vi "MainRT.vi"() -> ()   [LabVIEW 2018]
uses:
  Type Defs/The Motion Parameters.ctl
  Type Defs/G Code Command Cluster.ctl
  <vilib>/Motion/Express/_s/nimc.ex.clearFaults.clearFaults.axis.vi
  <vilib>/Motion/Express/_s/nimc.ex.power.power.axis.vi
  <vilib>/Motion/Express/_s/nimc.ex.read.readFaults.axis.vi
  <vilib>/Motion/BlockNode/FB.NIMotion.xnode
panel:
  in  "G Code File Path":path=path "c:/ni-rt/1cmQube.gcode"
  out "Ready":bool
  out "G Code Parser Progress":dbl(slide) scale=0.0..1.0
  out "Current Extruder Temp":dbl
  out "Current Bed Temp":dbl
  in  "Set Bed Temp":dbl
  in  "Monitor Stop":bool
  out "G Code Command Cluster":T1
  out "Faults":i32[][](array[numeric])
  in  "Motion Parameters":T2={"Timeout"=-1.0, "Blend Mode"=10551335, "Acceleration"=50.0, "Deceleration"=50.0, "Accel. Jerk"=500.0, "Decel. Jerk"=500.0, "Smoothing"=1000.0, "Last Blend"=TRUE, "Blend Delay"=0.0} {"Blend Delay" format="%#_13g"; "Smoothing" format="%#_13g"; "Decel. Jerk" format="%#_13g"; "Accel. Jerk" format="%#_13g"; "Deceleration" format="%#_13g"; "Acceleration" format="%#_13g"; "Blend Mode" items=["At Profile Complete"=10551335, "At Deceleration"=10551334, "After Delay"=10551336]}
  out "Error Out":errorcluster
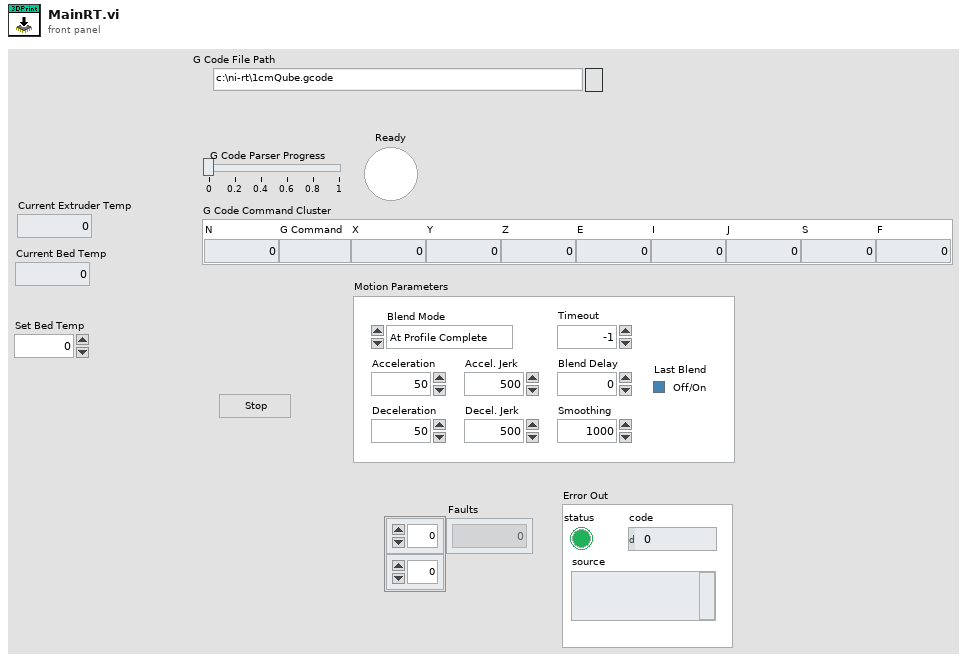
[diagram p1: front panel]
types:
  T1 = typedef "G Code Command Cluster.ctl" = cluster{"N":dbl, "G Command":string, "X":dbl, "Y":dbl, "Z":dbl, "E":dbl, "I":dbl, "J":dbl, "S":dbl, "F":dbl}
  T2 = typedef "The Motion Parameters.ctl" = cluster{"Timeout":dbl, "Blend Mode":i32, "Acceleration":dbl, "Deceleration":dbl, "Accel. Jerk":dbl, "Decel. Jerk":dbl, "Smoothing":dbl, "Last Blend":bool, "Blend Delay":dbl}
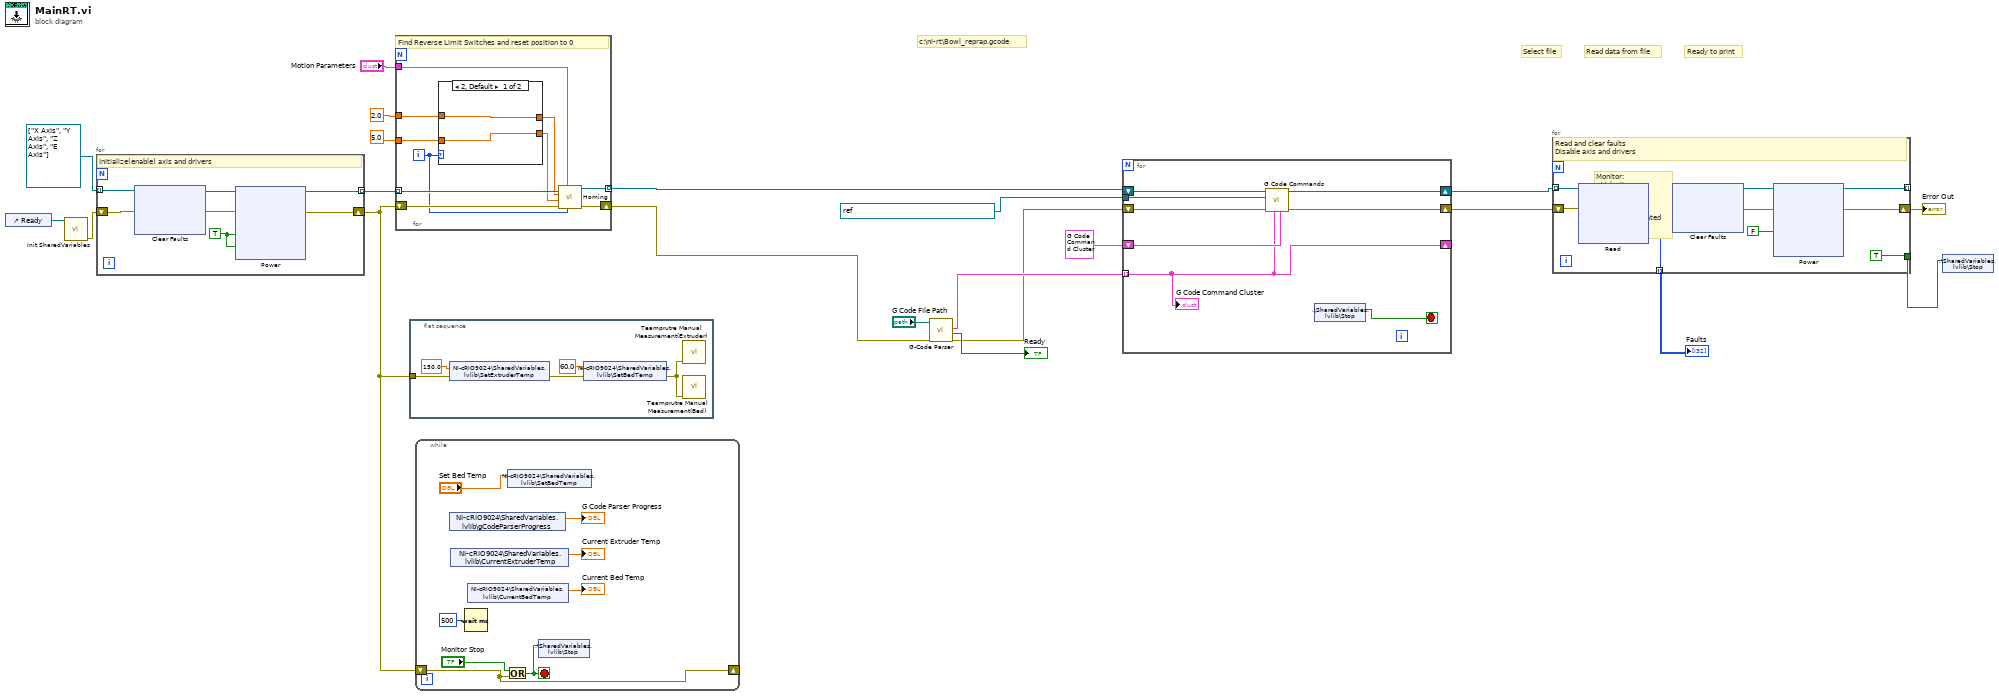
[diagram p0: block diagram]
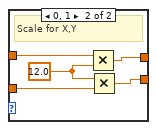
[diagram p2: hidden frame]
diagram:
  # "c:\\ni-rt\\Bowl_reprap.gcode"
  # "Ready to print"
  # "Select file"
  # "Monitor:\n- Velocity\n- Position\n- Faults\n- Temperature\n- Lines compleated"
  # "Execute G Code(for loop)"
  # "Read data from file"
  n1 = control-ref of="Ready"() -> (w1:refnum<vi>)
  n2 = call "Init SharedVariables.vi"("Boolean in"=w1) -> ("error out"=w4:errorcluster)  [unwired: 10 in]
  n3 = for {
    tunnel: refnum<k21>[] ["X Axis", "Y Axis", "Z Axis", "E Axis"] ("Axis Reference In") -> [w26] mode=indexing
    tunnel: [w25] -> w18 mode=indexing
    shift-right: [w23] -> w3
    shift-left: w4 -> [w22]
    w24 = TRUE ("enable axis")
    # "Initialize(enable) axis and drivers"
    n4 = xnode ("Clear Faults")("resource"=w26, "error in"=w22) -> ("resource out"=w28:refnum<k21>, "error out"=w27:errorcluster)
    n5 = xnode ("Power")("enable axis"=w24, "enable drive"=w24, "resource"=w28, "error in"=w27) -> ("resource out"=w25:refnum<k21>, "error out"=w23:errorcluster)
  }
  n6 = for {
    shift-right: [w49] -> w6
    shift-left: w3 -> [w50]
    tunnel: w18 -> [w48] mode=indexing
    tunnel: "Motion Parameters" -> [w44]
    tunnel: 5.0 ("Approach  Velocity") -> [w52]
    tunnel: 2.0 ("Search Velocity") -> [w51]
    tunnel: [w47] -> w5 mode=indexing
    i -> [w43]
    # "Find Reverse Limit Switches and reset position to 0"
    n7 = case shown="2, Default" w43 {
      tunnel: w52 -> [w54 w56]
      tunnel: [w54 w57] -> w46
      tunnel: w51 -> [w53 w58]
      tunnel: [w53 w59] -> w45
      frame 2, Default {
      }
      frame 0, 1 {
        w55 = 12.0 ("y")
        # "Scale for X,Y"
        n8 = Multiply(x=w58, y=w55) -> (x*y=w59:dbl)
        n9 = Multiply(x=w55, y=w56) -> (x*y=w57:dbl)
      }
    }
    n10 = call "Homing.vi"("Axis Index"=w43, "Motion Parameters"=w44, "Error In"=w50, "Approach  Velocity"=w46, "Search Velocity"=w45, "Axis Reference In"=w48) -> ("Error Out"=w49:errorcluster, "Axis Reference Out"=w47:refnum<k21>)  [unwired: 4 in]
  }
  n11 = flat-sequence {
    tunnel: w3 -> [w64]
    frame #0 {
      n12 = shared-variable "NI-cRIO9024\\SharedVariables.lvlib\\SetExtruderTemp"(150.0 ("Set Extruder Temp"), error in=w64) -> (error out=w63:errorcluster)
      n13 = shared-variable "NI-cRIO9024\\SharedVariables.lvlib\\SetBedTemp"(60.0 ("Set Bed Temp"), error in=w63) -> (error out=w62:errorcluster)
      n14 = call "Teamprutre Manual Measurement(Extruder).vi"("Error In"=w62) -> ()  [unwired: 10 in, 1 out]
      n15 = call "Teamprutre Manual Measurement(Bed).vi"("Error In"=w62) -> ()  [unwired: 10 in, 1 out]
    }
  }
  n16 = while {
    shift-right: [w72] -> _
    shift-left: w3 -> [w72]
    stop <- w70 stop-if-true
    n17 = shared-variable "NI-cRIO9024\\SharedVariables.lvlib\\gCodeParserProgress"() -> (→"G Code Parser Progress":dbl)  [unwired: 1 in, 1 out]
    n18 = shared-variable "NI-cRIO9024\\SharedVariables.lvlib\\CurrentExtruderTemp"() -> (→"Current Extruder Temp":dbl)  [unwired: 1 in, 1 out]
    n19 = Wait (ms)(milliseconds to wait=u32 500) -> ()  [unwired: 1 out]
    n20 = shared-variable "NI-cRIO9024\\SharedVariables.lvlib\\CurrentBedTemp"() -> (→"Current Bed Temp":dbl)  [unwired: 1 in, 1 out]
    n21 = Or(x="Monitor Stop", y=w72) -> (x .or. y?=w70:bool)
    n22 = shared-variable "NI-cRIO9024\\SharedVariables.lvlib\\SetBedTemp"("Set Bed Temp") -> ()  [unwired: 1 in, 1 out]
    n23 = shared-variable ".\\SharedVariables.lvlib\\Stop"(w70) -> ()  [unwired: 1 in, 1 out]
  }
  n24 = call "G-Code Parser.vi"("Error In"=w6, "G Code File Path"="G Code File Path") -> ("Error Out"=w7:errorcluster, "Ready"=→"Ready":bool, "G Code Commands"=w12:T1[])  [unwired: 7 in]
  n25 = for {
    tunnel: refnum<k21> "nism://NI-cRIO9024/Printer Space" ("Coordinate Space Reference In") -> [w78]
    shift-right: [w80] -> w15
    shift-left: w7 -> [w76]
    tunnel: w12 -> [w74] mode=indexing
    shift-right: [w74] -> _
    shift-left: T1 {"N"=0.0, "G Command"="", "X"=0.0, "Y"=0.0, "Z"=0.0, "E"=0.0, "I"=0.0, "J"=0.0, "S"=0.0, "F"=0.0} ("G Code Command Cluster") -> [w75]
    shift-right: [w79] -> w14
    shift-left: w5 -> [w77]
    stop <- w73 stop-if-true
    n26 = call "G Code Commands.vi"("Previous G Code"=w75, "Current G Code"=w74, "Error In"=w76, "Coordinate Space Reference In"=w78, "Axis Resources In"=w77) -> ("Error Out"=w80:errorcluster, "Axis Resources Out"=w79:refnum<k21>[])  [unwired: 4 in, 1 out]
    n27 = shared-variable ".\\SharedVariables.lvlib\\Stop"() -> (w73:bool)  [unwired: 1 in, 1 out]
    "G Code Command Cluster" <- w74
  }
  n28 = for {
    tunnel: [w89] -> _ mode=indexing
    shift-right: [w87] -> w17
    shift-left: w15 -> [w84]
    tunnel: [w83] -> w16 mode=indexing
    tunnel: w14 -> [w82] mode=indexing
    tunnel: [TRUE] -> w9
    w88 = FALSE ("enable axis")
    # "Read and clear faults \nDisable axis and drivers"
    n29 = xnode ("Read")("resource"=w82, "error in"=w84) -> ("fault code[] out"=w83:i32[], "resource out"=w86:refnum<k21>, "error out"=w85:errorcluster)  [unwired: 1 in, 1 out]
    n30 = xnode ("Clear Faults")("resource"=w86, "error in"=w85) -> ("resource out"=w91:refnum<k21>, "error out"=w90:errorcluster)
    n31 = xnode ("Power")("enable axis"=w88, "enable drive"=w88, "resource"=w91, "error in"=w90) -> ("resource out"=w89:refnum<k21>, "error out"=w87:errorcluster)
  }
  "Error Out" <- w17
  "Faults" <- w16
  n32 = shared-variable ".\\SharedVariables.lvlib\\Stop"(w9) -> ()  [unwired: 1 in, 1 out]
